vi "Calculate Clan.vi"(10 "Y":i32, 11 "X":i32) -> (3 "Clan":T1)   [LabVIEW 2015, in "Pinwheel.lvclass"]
uses:
  Pinwheel.lvclass
  Type Defs/Direction Enum.ctl
  Type Defs/SB Type Defs.lvlib
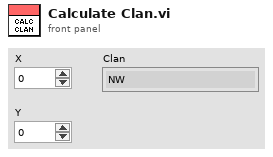
[diagram p1: front panel]
types:
  T1 = typedef "SB Type Defs.lvlib/Direction Enum.ctl" = enum16{"NW", "N", "NE", "E", "SE", "S", "SW", "W"}
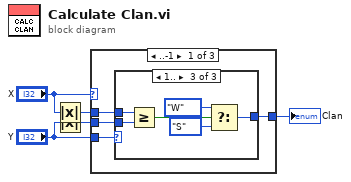
[diagram p0: block diagram]
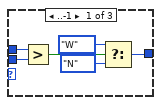
[diagram p2: hidden frame]
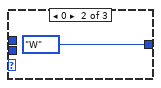
[diagram p3: hidden frame]
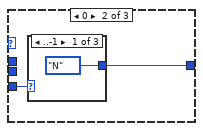
[diagram p4: hidden frame]
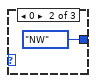
[diagram p5: hidden frame]
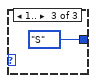
[diagram p6: hidden frame]
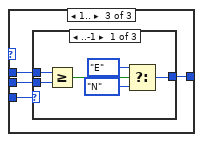
[diagram p7: hidden frame]
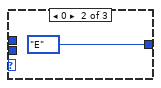
[diagram p8: hidden frame]
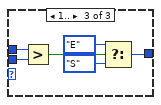
[diagram p9: hidden frame]
diagram:
  n1 = Absolute Value(x="X") -> (abs(x)=w2:i32)
  n2 = Absolute Value(x="Y") -> (abs(x)=w1:i32)
  n3 = case shown="..-1" "X" {
    tunnel: "Y" -> [w9 w24 w31]
    tunnel: [w8 w23 w30] -> w5
    tunnel: w2 -> [w7 _ w29]
    tunnel: w1 -> [w6 _ w28]
    frame ..-1 {
      n4 = case shown="1.." w9 {
        tunnel: [w10 Direction_Enum."W" ("Clan") w17] -> w8
        tunnel: w7 -> [w15 _ w22]
        tunnel: w6 -> [w14 _ w21]
        frame ..-1 {
          n5 = Greater?(x=w15, y=w14) -> (0:w13:bool)
          n6 = Select(t=Direction_Enum."W" ("Clan"), s=w13, f=Direction_Enum."N" ("Clan")) -> (s? t:f=w10:T1)
        }
        frame 0 {
        }
        frame 1.. {
          n7 = Greater Or Equal?(x=w22, y=w21) -> (x >= y?=w20:bool)
          n8 = Select(t=Direction_Enum."W" ("Clan"), s=w20, f=Direction_Enum."S" ("Clan")) -> (s? t:f=w17:T1)
        }
      }
    }
    frame 0 {
      n9 = case shown="..-1" w24 {
        tunnel: [Direction_Enum."N" ("Clan") Direction_Enum."NW" ("Clan") Direction_Enum."S" ("Clan")] -> w23
        frame ..-1 {
        }
        frame 0 {
        }
        frame 1.. {
        }
      }
    }
    frame 1.. {
      n10 = case shown="..-1" w31 {
        tunnel: [w32 Direction_Enum."E" ("Clan") w39] -> w30
        tunnel: w29 -> [w37 _ w44]
        tunnel: w28 -> [w36 _ w43]
        frame ..-1 {
          n11 = Greater Or Equal?(x=w37, y=w36) -> (x >= y?=w35:bool)
          n12 = Select(t=Direction_Enum."E" ("Clan"), s=w35, f=Direction_Enum."N" ("Clan")) -> (s? t:f=w32:T1)
        }
        frame 0 {
        }
        frame 1.. {
          n13 = Greater?(x=w44, y=w43) -> (0:w42:bool)
          n14 = Select(t=Direction_Enum."E" ("Clan"), s=w42, f=Direction_Enum."S" ("Clan")) -> (s? t:f=w39:T1)
        }
      }
    }
  }
  "Clan" <- w5
